vi "Dual Single Gauge - Example 2.vi"(8 "error in (no error)":errorcluster caption="Fehler (Eingang, kein Fehler)", 11 "input refnum":refnum<visa-resource-name> caption="Eingang (Referenz)") -> (0 "error out":errorcluster, 1 "Status Sensor 2":i32(ring) items=["data OK", "underrange", "overrange", "sensor error", "sensor off", "no sensor", "ID error"], 2 "Status Sensor 1":i32(ring) items=["data OK", "underrange", "overrange", "sensor error", "sensor off", "no sensor", "ID error"], 3 "Pressure Sensor 2":dbl format="%.3e", 5 "Pressure Sensor 1":dbl format="%.3e")   [LabVIEW 2013, in "Dual Gauge.lvlib"]
uses:
  Dual Gauge.lvlib
panel:
  out "Get Calibration factor 2":dbl=0.000753 format="%.3f"
  out "Get Calibration factor 1":dbl=0.000753 format="%.3f"
  out "Sensor 2 Get 2":i8(ring)=1 items=["fast", "normal", "slow"]
  out "Sensor 1 Get 2":i8(ring)=1 items=["fast", "normal", "slow"]
  out "Sensor 2 Get":u8(ring)=3 items=["0.01 mbar", "0.1 mbar", "1 mbar", "10 mbar", "100 mbar", "1000 mbar", "2 bar", "5 bar", "10 bar", "50 bar"]
  out "Sensor 1 Get":u8(ring)=3 items=["0.01 mbar", "0.1 mbar", "1 mbar", "10 mbar", "100 mbar", "1000 mbar", "2 bar", "5 bar", "10 bar", "50 bar"]
  out "Sensor 2 Set":u8(ring) items=["no change / no sensor", "off", "automatic", "on"]
  out "Sensor 1 Set":u8(ring) items=["no change / no sensor", "off", "automatic", "on"]
  out "Sensor 2":string
  out "Sensor 1":string
  in  "Unit Set":i8(ring) items=["mbar / bar", "Torr", "Pascal"]
  out "Unit Get":i8(ring) items=["mbar / bar", "Torr", "Pascal"]
  in  "W/R":bool
  out "Programversion":string
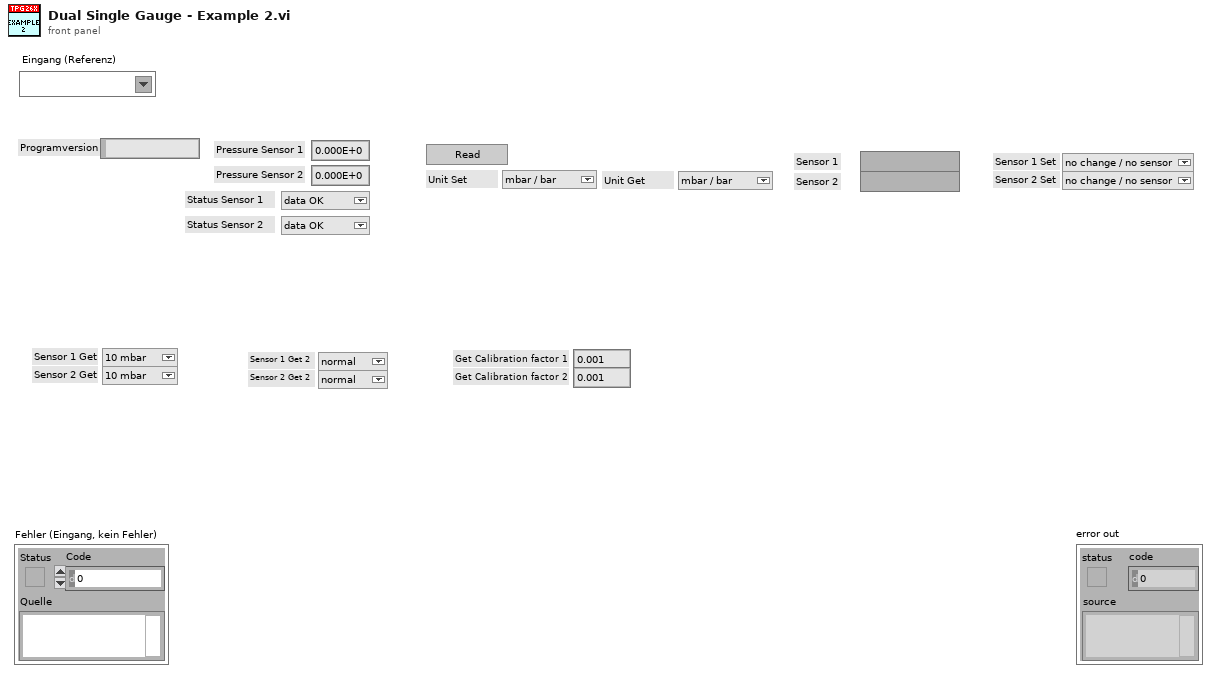
[diagram p1: front panel]
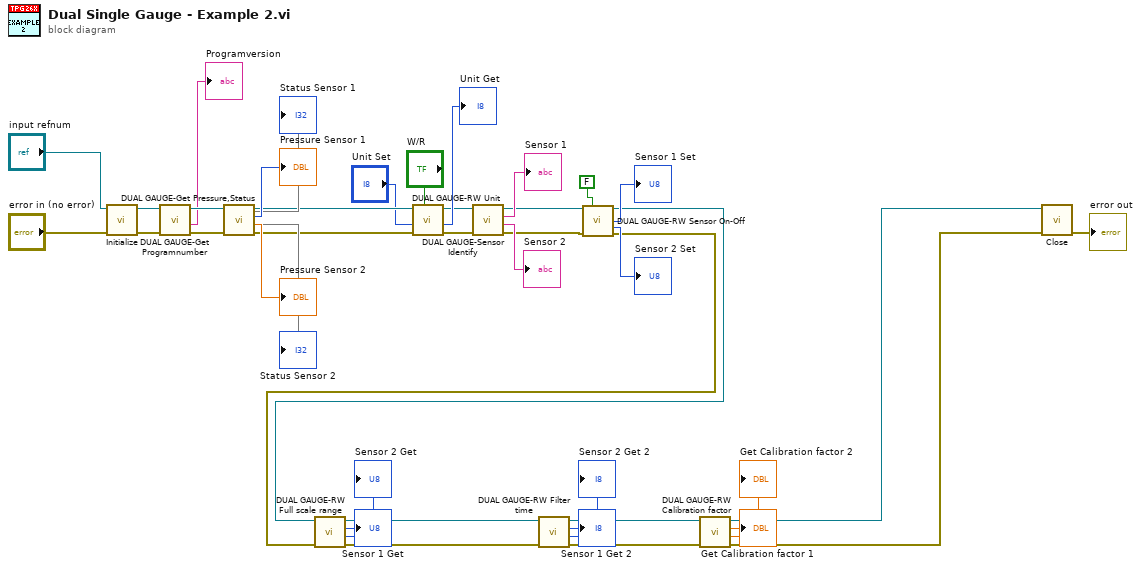
[diagram p0: block diagram]
diagram:
  n1 = call "Initialize.vi"("error in (no error)"="error in (no error)", "input refnum"="input refnum") -> ("Cluster (Ausgang)"=w31:errorcluster, "Referenz out"=w33:refnum<visa-resource-name>)  [unwired: 8 in]
  n2 = call "DUAL GAUGE-Get Programnumber.vi"("Fehler (Eingang)"=w31, "Referenz in"=w33) -> ("Cluster (Ausgang)"=w30:errorcluster, "Programversion"=→"Programversion":string, "Referenz out"=w32:refnum<visa-resource-name>)  [unwired: 7 in]
  n3 = call "DUAL GAUGE-Get Pressure,Status.vi"("Fehler (Eingang)"=w30, "Referenz in"=w32) -> ("Cluster (Ausgang)"=w27:errorcluster, "Pressure"=→"Pressure Sensor 2":dbl, "Status"=→"Pressure Sensor 1":i32, "Referenz out"=w28:refnum<visa-resource-name>, 4:→"Status Sensor 2", 5:→"Status Sensor 1")  [unwired: 4 in]
  n4 = call "DUAL GAUGE-RW Unit.vi"("W/R"="W/R", "Fehler (Eingang)"=w27, "Unit Set"="Unit Set", "Referenz in"=w28) -> ("Cluster (Ausgang)"=w22:errorcluster, "Unit Get"=→"Unit Get":i8, "Referenz out"=w23:refnum<visa-resource-name>)  [unwired: 5 in]
  n5 = call "DUAL GAUGE-Sensor Identify.vi"("Fehler (Eingang)"=w22, "Referenz in"=w23) -> ("Cluster (Ausgang)"=w18:errorcluster, "Sensor 2"=→"Sensor 2":string, "Sensor 1"=→"Sensor 1":string, "Referenz out"=w19:refnum<visa-resource-name>)  [unwired: 6 in]
  n6 = call "DUAL GAUGE-RW Sensor On-Off.vi"("Referenz in"=w19, "W/R"=FALSE, "Fehler (Eingang)"=w18) -> ("Referenz out"=w12:refnum<visa-resource-name>, "Sensor 1 Set"=→"Sensor 1 Set":u8, "Sensor 2 Set"=→"Sensor 2 Set":u8, "Cluster (Ausgang)"=w8:errorcluster)  [unwired: 9 in]
  n7 = call "DUAL GAUGE-RW Full scale range.vi"("Fehler (Eingang)"=w8, "Referenz in"=w12) -> ("Cluster (Ausgang)"=w10:errorcluster, "Sensor 2 Get"=→"Sensor 2 Get":u8, "Sensor 1 Get"=→"Sensor 1 Get":u8, "Referenz out"=w14:refnum<visa-resource-name>)  [unwired: 6 in]
  n8 = call "DUAL GAUGE-RW Filter time.vi"("Fehler (Eingang)"=w10, "Referenz in"=w14) -> ("Cluster (Ausgang)"=w9:errorcluster, "Sensor 2 Get"=→"Sensor 2 Get 2":i8, "Sensor 1 Get"=→"Sensor 1 Get 2":i8, "Referenz out"=w13:refnum<visa-resource-name>)  [unwired: 6 in]
  n9 = call "DUAL GAUGE-RW Calibration factor.vi"("Fehler (Eingang)"=w9, "Referenz in"=w13) -> ("Cluster (Ausgang)"=w7:errorcluster, "Get Calibration factor 2"=→"Get Calibration factor 2":dbl, "Get Calibration factor 1"=→"Get Calibration factor 1":dbl, "Referenz out"=w11:refnum<visa-resource-name>)  [unwired: 6 in]
  n10 = call "Close.vi"("error in (no error)"=w7, "VISA resource name"=w11) -> ("error out"=→"error out":errorcluster)  [unwired: 9 in]
